vi "Apply Style - Simple Dialog.vi"(4 "button refs":refnum<vi>[](array[refnum]), 7 "title ref":refnum<vi>, 8 "error in":errorcluster, 9 "message ref":refnum<vi>, 10 "pop up ref":refnum<vi>, 11 "Theme in":refnum<class "Theme.lvclass">) -> (0 "error out":errorcluster, 3 "Theme out":refnum<class "Theme.lvclass">)   [LabVIEW 2021, in "Theme.lvclass"]
doc: "Apply the style to the message pop up : format the header, background, and message box\n\n<b>Code Developed By:</b>\nTechnology Service Corporation\n1983 S Liberty Drive\nBloomington, IN 47403\nPhone: 812 558-7100\nwww.tsc.com/atcs\n\nDeveloper:\nDaniel Coons"
uses:
  Theme.lvclass
  <vilib>/Utility/miscctls.llb/LVSelectionTypeDef.ctl
  Theme.lvclass/Theme.ctl
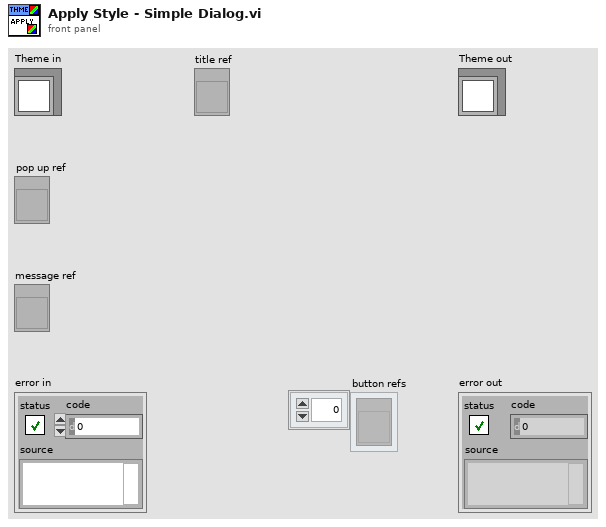
[diagram p1: front panel]
types:
  T1 = typedef "LVSelectionTypeDef.ctl" = cluster{"Selection Start":u32, "Selection End":u32}
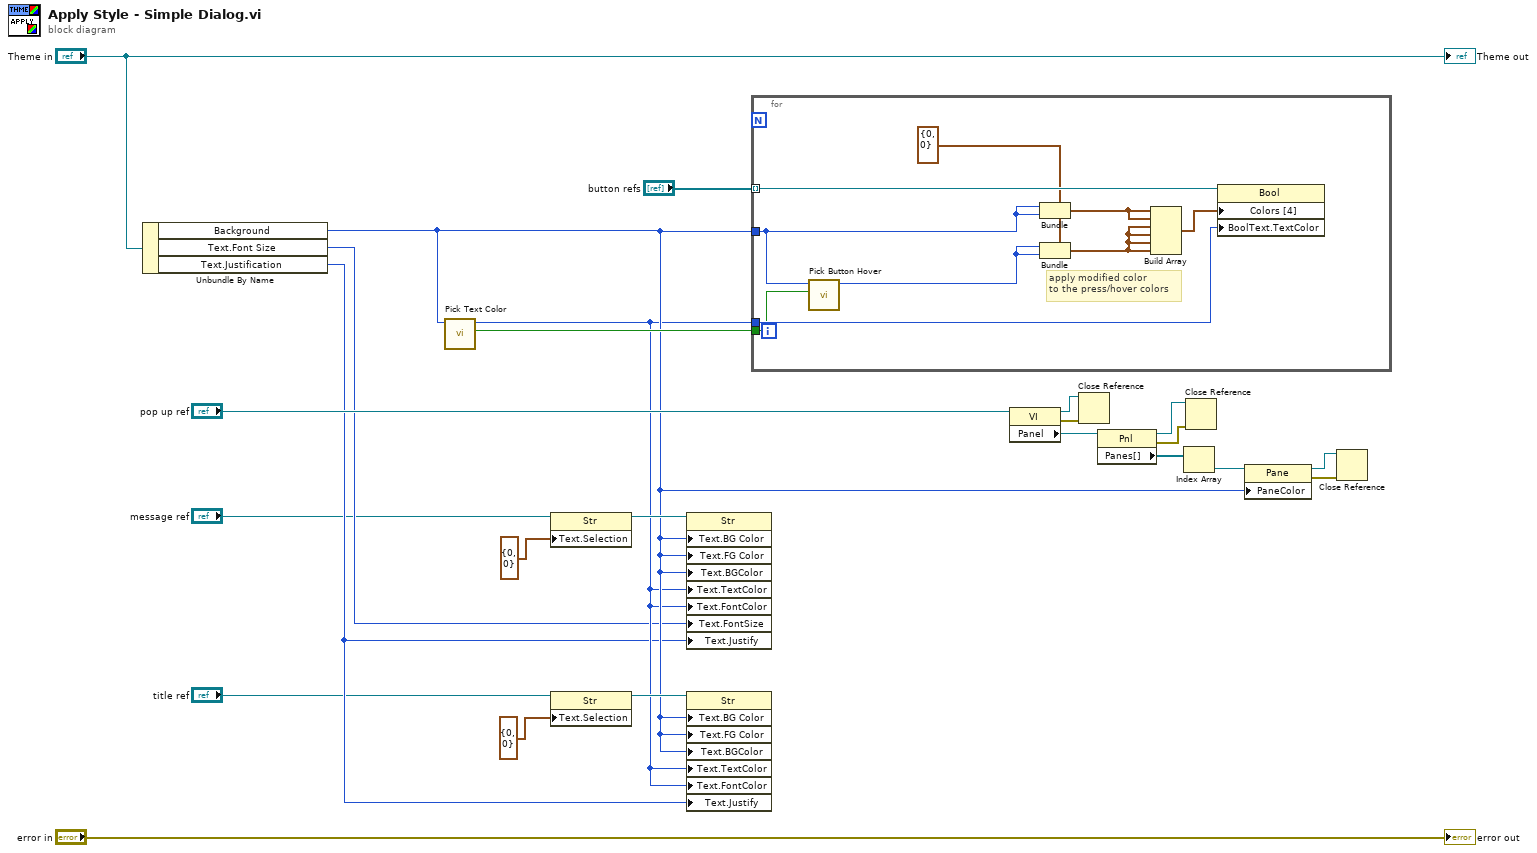
[diagram p0: block diagram]
diagram:
  n1 = Unbundle By Name("Theme in") -> ("Background"=w6:u32, "Text.Font Size"=w4:u32, "Text.Justification"=w3:enum16{"Left", "Center", "Right"})
  n2 = call "Pick Text Color.vi"("color"=w6) -> ("light?"=w11:bool, "text"=w5:u32)  [unwired: 9 in]
  n3 = property class="Str"(reference="message ref", "Text.Selection"=T1 {"Selection Start"=0, "Selection End"=0}) -> (reference out=w10:refnum<vi>)  [unwired: 1 in, 1 out]
  n4 = property class="Str"(reference="title ref", "Text.Selection"=T1 {"Selection Start"=0, "Selection End"=0}) -> (reference out=w7:refnum<vi>)  [unwired: 1 in, 1 out]
  n5 = property on="Property Node" class="Str"(reference=w10, "Text.BG Color"=w6, "Text.FG Color"=w6, "Text.BGColor"=w6, "Text.TextColor"=w5, "Text.FontColor"=w5, "Text.FontSize"=w4, "Text.Justify"=w3) -> ()  [unwired: 1 in, 2 out]
  n6 = property on="Property Node" class="Str"(reference=w7, "Text.BG Color"=w6, "Text.FG Color"=w6, "Text.BGColor"=w6, "Text.TextColor"=w5, "Text.FontColor"=w5, "Text.Justify"=w3) -> ()  [unwired: 1 in, 2 out]
  n7 = for {
    tunnel: "button refs" -> [w32] mode=indexing
    tunnel: w5 -> [w31]
    tunnel: w6 -> [w27]
    tunnel: w11 -> [w26]
    w29 = cluster{u32, u32} {0, 0}
    # "apply modified color \nto the press/hover colors"
    n8 = call "Pick Button Hover.vi"("light?"=w26, "Background"=w27) -> ("Color"=w25:u32)  [unwired: 9 in]
    n9 = Bundle(cluster=w29, w27, w27) -> (w30:cluster{u32, u32})
    n10 = Bundle(cluster=w29, w25, w25) -> (w28:cluster{u32, u32})
    n11 = Build Array(w30, w30, w28, w28, w28, w28) -> (w33:cluster{u32, u32}[])
    n12 = property on="Property Node" class="Bool"(reference=w32, "Colors [4]"=w33, "BoolText.TextColor"=w31) -> ()  [unwired: 1 in, 2 out]
  }
  n13 = property class="VI"(reference="pop up ref") -> (reference out=w13:refnum<vi>, error out=w21:errorcluster, "Panel"=w20:refnum<vi>)  [unwired: 1 in]
  n14 = Close Reference(reference=w13, error in (no error)=w21) -> ()  [unwired: 1 out]
  n15 = property class="Pnl"(reference=w20) -> (reference out=w14:refnum<vi>, error out=w22:errorcluster, "Panes[]"=w19:refnum<vi>[])  [unwired: 1 in]
  n16 = Index Array(array=w19) -> (element=w18:refnum<vi>)  [unwired: 1 in]
  n17 = Close Reference(reference=w14, error in (no error)=w22) -> ()  [unwired: 1 out]
  n18 = property class="Pane"(reference=w18, "PaneColor"=w6) -> (reference out=w15:refnum<vi>, error out=w23:errorcluster)  [unwired: 1 in]
  n19 = Close Reference(reference=w15, error in (no error)=w23) -> ()  [unwired: 1 out]
  "error out" <- "error in"
  "Theme out" <- "Theme in"
